vi "LookAheadPoint.vi"(6 "Reset":bool, 8 "Robot":cluster{"x":dbl, "y":dbl}, 9 "Spacing":dbl, 10 "LookAhead":dbl, 11 "Path":cluster{"x":dbl, "y":dbl}[](array[cluster])) -> (2 "LookaheadIndex":i32, 3 "Point":cluster{"x":dbl, "y":dbl})   [LabVIEW 2017]
doc: "Finds the lookahead point given a path and the current location of the robot."
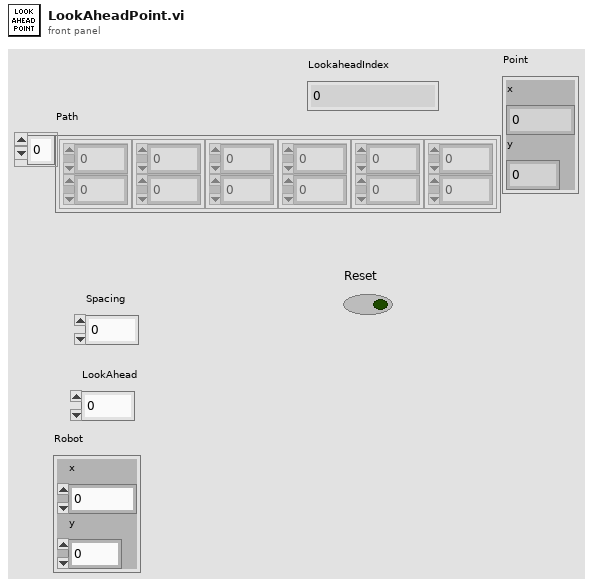
[diagram p1: front panel]
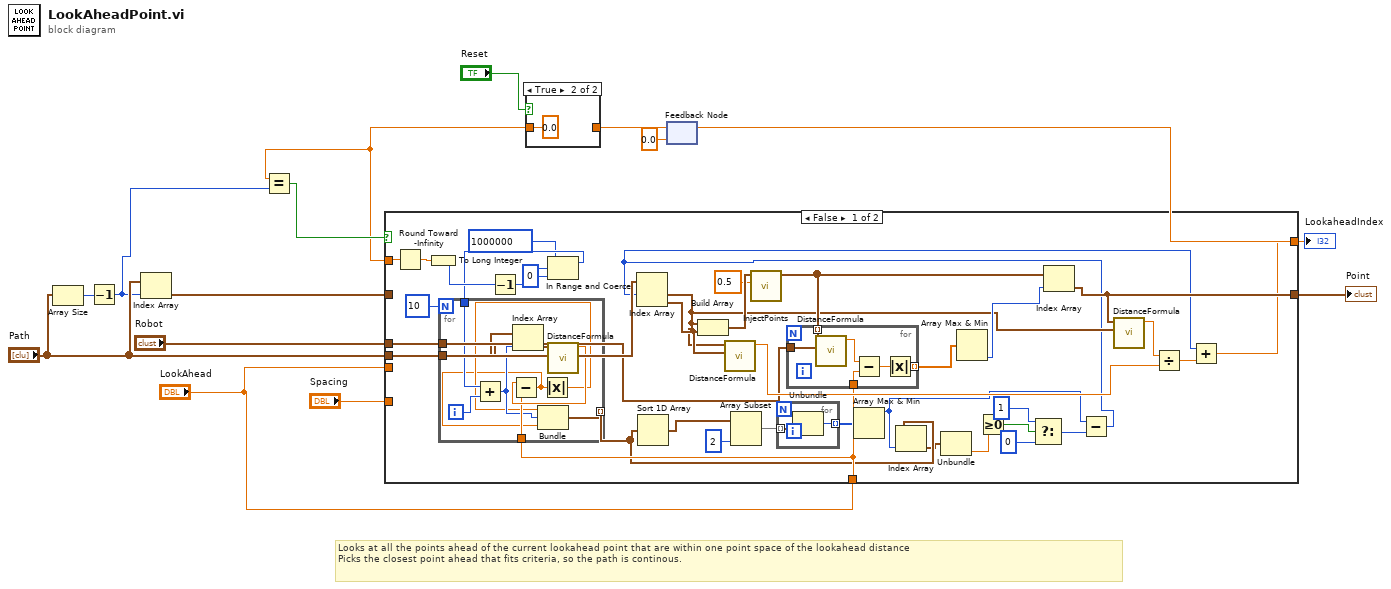
[diagram p0: block diagram]
diagram:
  # "Looks at all the points ahead of the current lookahead point that are within one point space of the lookahead distance\nPicks the closest point ahead that fits criteria, so the path is continous."
  n1 = Array Size(array="Path") -> (size(s)=w13:i32)
  n2 = Decrement(x=w13) -> (x-1=w5:i32)
  n3 = Index Array(array="Path", index=w5) -> (element=w11:cluster{"x":dbl, "y":dbl})
  n4 = feedback #1(0.0) -> (w8:dbl)
  n5 = case shown="True" "Reset" {
    tunnel: w8 -> [w15 _]
    tunnel: [w15 0.0] -> w3
    frame False {
    }
    frame True {
    }
  }
  n6 = Equal?(x=w3, y=w5) -> (x = y?=w4:bool)
  n7 = case shown="False" w4 {
    tunnel: "LookAhead" -> [_ _]
    tunnel: [w44 w73] -> w14
    tunnel: "Path" -> [w37 _]
    tunnel: "Robot" -> [w36 _]
    tunnel: [w39 w72] -> w7
    tunnel: w11 -> [_ w73]
    tunnel: "Spacing" -> [_ _]
    tunnel: w3 -> [w46 w72]
    tunnel: "LookAhead" -> [w35 _]
    frame False {
      n8 = Round Toward -Infinity(1:w46) -> (0:w47:dbl)
      n9 = To Long Integer(number=w47) -> (32bit integer=w21:i32)
      n10 = Decrement(x=w21) -> (x-1=w20:i32)
      n11 = In Range and Coerce(upper limit=1000000, x=w20, lower limit=0) -> (coerced(x)=w18:i32)  [unwired: 1 out]
      n12 = for {
        N: 10 -> [_]
        tunnel: w18 -> [w64]
        tunnel: w37 -> [w63]
        tunnel: w36 -> [w61]
        tunnel: w35 -> [w59]
        tunnel: [w57] -> w30 mode=indexing
        i -> [w65]
        n13 = Add(x=w64, y=w65) -> (x+y=w58:i32)
        n14 = Index Array(array=w63, index=w58) -> (element=w62:cluster{"x":dbl, "y":dbl})
        n15 = call "DistanceFormula.vi"("Point 2"=w61, "Point 1"=w62) -> ("Distance"=w60:dbl)  [unwired: 9 in]
        n16 = Subtract(x=w60, y=w59) -> (x-y=w55:dbl)
        n17 = Absolute Value(x=w55) -> (abs(x)=w56:dbl)
        n18 = Bundle(w56, w58, w55) -> (w57:cluster{dbl, i32, dbl})  [unwired: 1 in]
      }
      n19 = Sort 1D Array(array=w30) -> (sorted array=w34:cluster{dbl, i32, dbl}[])
      n20 = Array Subset(array=w34, length=2) -> (w32:cluster{dbl, i32, dbl}[])  [unwired: 1 in]
      n21 = for {
        tunnel: w32 -> [w54] mode=indexing
        tunnel: [w53] -> w31 mode=indexing
        n22 = Unbundle(w54) -> (w53:i32)  [unwired: 2 out]
      }
      n23 = Array Max & Min(array=w31) -> (max value=w23:i32)  [unwired: 3 out]
      n24 = Index Array(array=w30, index=w23) -> (element=w29:cluster{dbl, i32, dbl})
      n25 = Unbundle(w29) -> (w28:dbl)  [unwired: 2 out]
      n26 = Greater Or Equal To 0?(x=w28) -> (x >= 0?=w27:bool)
      n27 = Select(t=1 ("length"), s=w27, f=0 ("length")) -> (s? t:f=w24:i32)
      n28 = Subtract(x=w23, y=w24) -> (x-y=w22:i32)
      n29 = Index Array(array=w37, index #1=w22) -> (element #1=w43:cluster{"x":dbl, "y":dbl}, element #2=w45:cluster{"x":dbl, "y":dbl})  [unwired: 1 in]
      n30 = Build Array(w43, w45) -> (w52:cluster{"x":dbl, "y":dbl}[])
      n31 = call "DistanceFormula.vi"("Point 2"=w45, "Point 1"=w43) -> ("Distance"=w41:dbl)  [unwired: 9 in]
      n32 = call "InjectPoints.vi"("Spacing"=0.5, "Path"=w52) -> ("Path out"=w48:cluster{dbl, dbl}[])  [unwired: 9 in]
      n33 = for {
        tunnel: w48 -> [w69] mode=indexing
        tunnel: w36 -> [w68]
        tunnel: w35 -> [w67]
        tunnel: [w66] -> w50 mode=indexing
        n34 = call "DistanceFormula.vi"("Point 2"=w68, "Point 1"=w69) -> ("Distance"=w70:dbl)  [unwired: 9 in]
        n35 = Subtract(x=w70, y=w67) -> (x-y=w71:dbl)
        n36 = Absolute Value(x=w71) -> (abs(x)=w66:dbl)
      }
      n37 = Array Max & Min(array=w50) -> (min index (indices)=w49:i32)  [unwired: 3 out]
      n38 = Index Array(array=w48, index=w49) -> (element=w44:cluster{dbl, dbl})
      n39 = call "DistanceFormula.vi"("Point 2"=w43, "Point 1"=w44) -> ("Distance"=w42:dbl)  [unwired: 9 in]
      n40 = Divide(x=w42, y=w41) -> (x/y=w40:dbl)
      n41 = Add(x=w22, y=w40) -> (x+y=w39:dbl)
    }
    frame True {
    }
  }
  "Point" <- w14
  "LookaheadIndex" <- w7
  n42 = feedback-in #1(w7) -> ()
